vi "DIAG_STM Write Meta Data (TCP Ref).vi"(6 "Options":T1={"Ignore Timeout Error"=TRUE, "timeout ms (1000)"=1000}, 7 "Meta data":T2[](array[typedef]), 8 "error in":errorcluster, 11 "connection ID":refnum<k5>) -> (0 "error out":errorcluster, 3 "Connection Info Out":T3)   [LabVIEW 2015, in "Diagnostics Addon Engine.lvlib"]
doc: "Use this VI to transmit the meta data cluster to a remote computer. Sending the meta data to another computer helps maintainability since the data resides only on one side and it is shared to other computers at run time."
uses:
  Diagnostics Addon Engine.lvlib
  stm_TCP Connection Info.ctl
  _SubVIs/stm_MetaDataElement.ctl
  stm_TCP Write Options.ctl
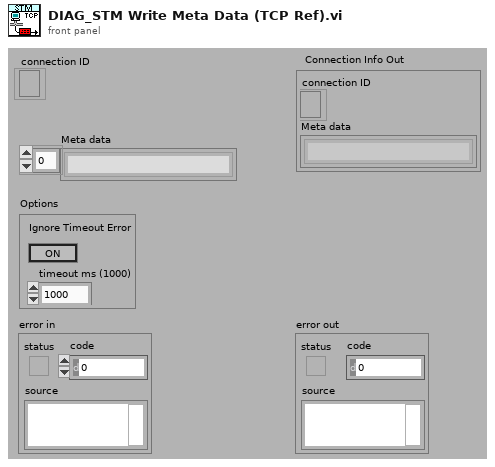
[diagram p1: front panel]
types:
  T1 = typedef "Diagnostics Addon Engine.lvlib/stm_TCP Write Options.ctl" = cluster{"Ignore Timeout Error":bool, "timeout ms (1000)":i32}
  T2 = typedef "Diagnostics Addon Engine.lvlib/stm_MetaDataElement.ctl" = string
  T3 = typedef "Diagnostics Addon Engine.lvlib/stm_TCP Connection Info.ctl" = cluster{"connection ID":refnum<k5>, "Meta data":T2[]}
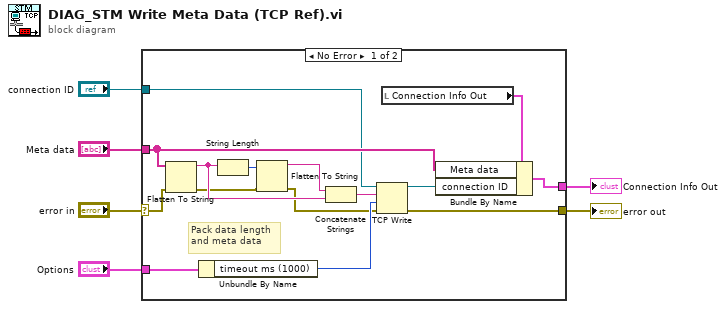
[diagram p0: block diagram]
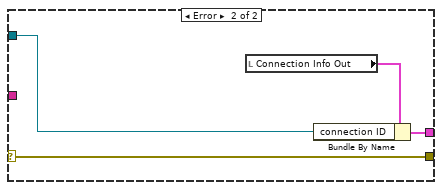
[diagram p2: hidden frame]
diagram:
  n1 = case shown="No Error" "error in" {
    selector: "error in" -> [w11 w25]
    tunnel: [w13 w23] -> w6
    tunnel: "connection ID" -> [w8 w22]
    tunnel: "Meta data" -> [w12 _]
    tunnel: [w21 w25] -> w4
    tunnel: "Options" -> [w16 _]
    frame No Error {
      # "Pack data length\nand meta data"
      n2 = Flatten To String(anything=w12, error in (no error)=w11) -> (data string=w17:string, error out=w10:errorcluster)  [unwired: 3 out]
      n3 = Unbundle By Name(w16) -> ("timeout ms (1000)"=w15:i32)
      n4 = String Length(string=w17) -> (length=w20:i32)
      n5 = Flatten To String(anything=w20, error in (no error)=w10) -> (data string=w19:string, error out=w9:errorcluster)  [unwired: 3 out]
      n6 = Concatenate Strings(w19, w17) -> (w18:string)
      n7 = TCP Write(connection ID=w8, data in=w18, error in (no error)=w9, 9:w15) -> (connection ID out=w14:refnum<k5>, error out=w21:errorcluster)  [unwired: 1 out]
      n8 = local read "Connection Info Out"() -> (w7:T3)
      n9 = Bundle By Name(cluster=w7, "Meta data"=w12, "connection ID"=w14) -> (w13:T3)
    }
    frame Error {
      n10 = local read "Connection Info Out"() -> (w24:T3)
      n11 = Bundle By Name(cluster=w24, "connection ID"=w22) -> (w23:T3)
    }
  }
  "Connection Info Out" <- w6
  "error out" <- w4
